vi "02. Native MQTT Data Consumer.vi"() -> ()   [LabVIEW 2019]
uses:
  <vilib>/LabVIEW Open Source Project/MQTT Control Packets/Control Packets/ControlPacket/ControlPacket.lvclass/ControlPacket.ctl
  48b0a82f-0a40-4110-a44a-7236f563c430.vi
  <vilib>/LabVIEW Open Source Project/MQTT Control Packets/Control Packets/PUBLISH/PUBLISH.lvclass
  C:/Program Files (x86)/National Instruments/LabVIEW 2019/vi.lib/LabVIEW Open Source Project/MQTT Control Packets/Control Packets/ControlPacket/ControlPacket.lvclass
  <vilib>/JDP Science/JSONtext/JSON text to Variant.vi
  <vilib>/JDP Science/JSONtext/LVClass Serializer/JSONtext LVClass Serializer.lvclass
  <vilib>/LabVIEW Open Source Project/MQTT Control Packets/Control Packets/ControlPacket/ControlPacket.lvclass
panel:
  out "parsing error":errorcluster
  out "Waveform Chart":dbl(graph)
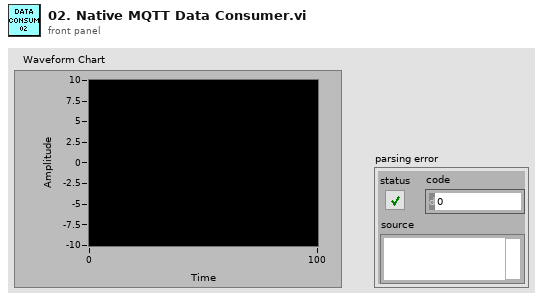
[diagram p1: front panel]
types:
  T1 = typedef "Actor Private Data.ctl" = cluster{"Client":refnum<class "Client.lvclass">, "QualifiedName":string, "EventReg":refnum<event-registration>, "Private Events":T2}
  T2 = typedef "Actor Private Events -- cluster.ctl" = cluster{"Stop":refnum<user-event>, "Subscribe":refnum<user-event>, "Unsubscribe":refnum<user-event>, "publish":refnum<user-event>}
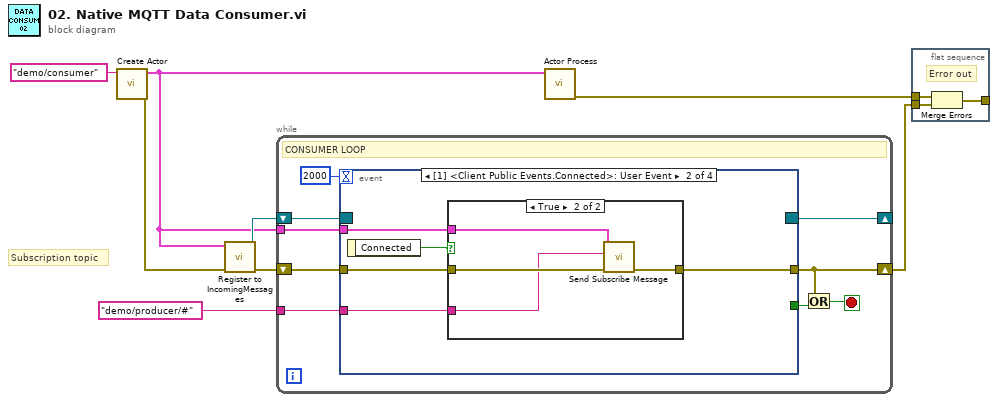
[diagram p0: block diagram]
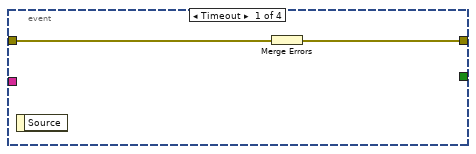
[diagram p2: hidden frame]
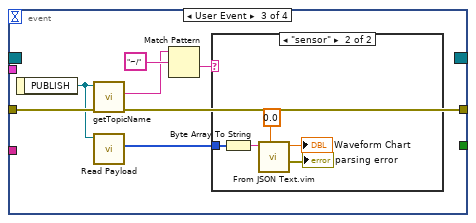
[diagram p4: hidden frame]
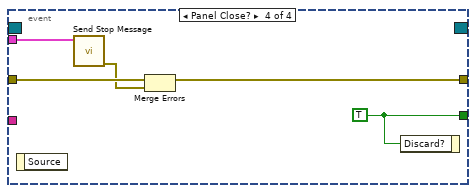
[diagram p6: hidden frame]
diagram:
  # "Subscription topic"
  n1 = call "Create Actor.vi"("QualifiedName"="demo/consumer") -> ("error out"=w7:errorcluster, "Actor Class"=w5:T1)  [unwired: 9 in]
  n2 = call "Register to IncomingMessages.vi"("error in"=w7, "Actor Class"=w5) -> ("error out"=w4:errorcluster, "Incoming Messages"=w6:refnum<event-registration>)  [unwired: 8 in]
  n3 = while {
    tunnel: w5 -> [w15]
    shift-right: [w12] -> _
    shift-left: w6 -> [w13]
    shift-right: [w10] -> w3
    shift-left: w4 -> [w11]
    tunnel: "demo/producer/#" ("QualifiedName") -> [w9]
    stop <- w16 stop-if-true
    # "CONSUMER LOOP"
    n4 = event shown="[1] <Client Public Events.Connected>: User Event" {
      selector: w13 -> [_ _ _ _]
      dyn-events: [_ _ _ _] -> w12
      timeout: 2000 -> [_ _ _ _]
      tunnel: [_ _ _ w46] -> w17
      tunnel: w15 -> [_ w22 _ w45]
      tunnel: [w18 w23 w35 w42] -> w10
      tunnel: w11 -> [w19 w24 w36 w44]
      tunnel: w9 -> [_ w20 _ _]
      event Timeout {
        n5 = event-data() -> ()  [unwired: 1 in, 1 out]
        n6 = Merge Errors(w19) -> (w18:errorcluster)
      }
      event User Event {
        n7 = event-data() -> ("Connected"=w21:bool)  [unwired: 1 in]
        n8 = case shown="True" w21 {
          tunnel: w24 -> [w25 w29]
          tunnel: [w25 w28] -> w23
          tunnel: w22 -> [_ w27]
          tunnel: w20 -> [_ w26]
          frame False {
          }
          frame True {
            n9 = call "Send Subscribe Message.vi"("error in"=w29, "Topic"=w26, "Actor Class"=w27) -> ("error out"=w28:errorcluster)  [unwired: 8 in]
          }
        }
      }
      event User Event {
        n10 = event-data() -> ("PUBLISH"=w31:refnum<class "PUBLISH.lvclass">)  [unwired: 1 in]
        n11 = call <vilib>:"getTopicName.vi"("error in (no error)"=w36, "PUBLISH in"=w31) -> ("error out"=w35:errorcluster, "Topic"=w33:string)  [unwired: 7 in, 1 out]
        n12 = call <vilib>:"Read Payload.vi"("ControlPacket in"=w31) -> ("Payload"=w30:u8[])  [unwired: 9 in, 1 out]
        n13 = Match Pattern(string=w33, regular expression="~/" ("QualifiedName")) -> (after substring=w32:string)  [unwired: 1 in, 3 out]
        n14 = case shown="\"sensor\"" w32 {
          tunnel: w30 -> [_ w41]
          frame Default {
          }
          frame "sensor" {
            n15 = Byte Array To String(unsigned byte array=w41) -> (string=w40:string)
            n16 = call "From JSON Text.vim"("Data Type and Default Value"=0.0, "JSON"=w40) -> ("error out"=→"parsing error":errorcluster, "Data out"=→"Waveform Chart":dbl)  [unwired: 8 in]
          }
        }
      }
      event Panel Close? {
        w46 = TRUE ("Discard?")
        n17 = event-data() -> ()  [unwired: 1 in, 1 out]
        n18 = call "Send Stop Message.vi"("Actor Class"=w45) -> ("error out"=w43:errorcluster)  [unwired: 10 in]
        n19 = Merge Errors(w44, w43) -> (w42:errorcluster)
        n20 = event-data("Discard?"=w46) -> ()  [unwired: 1 in, 1 out]
      }
    }
    n21 = Or(x=w10, y=w17) -> (x .or. y?=w16:bool)
  }
  n22 = call "Actor Process.vi"("Actor Class"=w5) -> ("error out"=w2:errorcluster)  [unwired: 10 in]
  n23 = flat-sequence {
    tunnel: w2 -> [w49]
    tunnel: w3 -> [w48]
    tunnel: [w47] -> _
    frame #0 {
      # "Error out"
      n24 = Merge Errors(w49, w48) -> (w47:errorcluster)
    }
  }
